vi "Set Initialization Data - TCP Send.vi"(8 "error in":errorcluster, 11 "Network End Point in":refnum<class "Network End Point.lvclass">) -> (0 "error out":errorcluster, 3 "Network End Point out":refnum<class "Network End Point.lvclass">)   [LabVIEW 2020, in "Network End Point.lvclass"]
doc: "Sets the initialization data of a statically linked subWorker."
uses:
  Network End Point.lvclass
  C:/Program Files (x86)/National Instruments/LabVIEW 2020/vi.lib/addons/_Workers/Library/Classes/Worker/Worker.lvclass
  TCP Send/Initialization Data.ctl
  <vilib>/addons/_Workers/Library/Classes/Message Queue/Message Queue.lvclass
  Network End Point.lvclass/Network End Point.ctl
  TCP Send/TCP Send.lvclass
  <vilib>/addons/_Workers/Library/Classes/Worker/Worker.lvclass
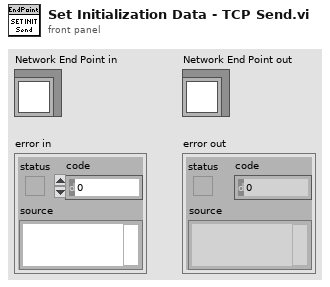
[diagram p1: front panel]
types:
  T1 = typedef "TCP Send.lvclass/Initialization Data.ctl" = cluster{"String":string, "connection ID":refnum<k5>, "End Point":refnum<class "Message Queue.lvclass">}
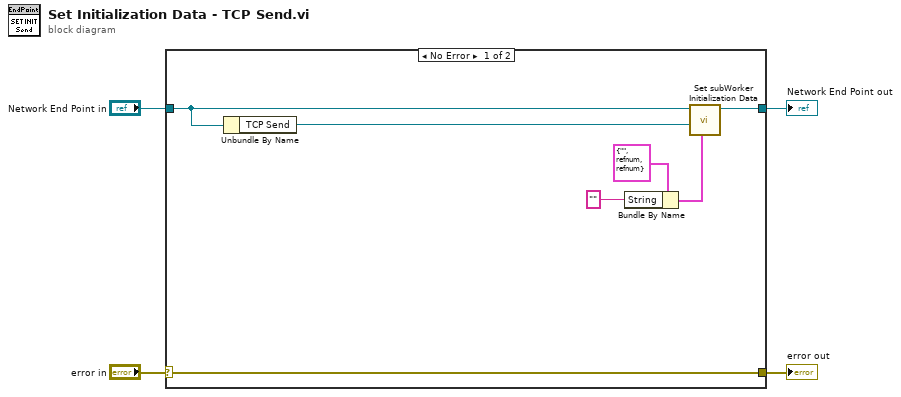
[diagram p0: block diagram]
diagram:
  n1 = case shown="No Error" "error in" {
    selector: "error in" -> [w11 w13]
    tunnel: [w11 w13] -> w3
    tunnel: [w9 w12] -> w2
    tunnel: "Network End Point in" -> [w8 w12]
    frame No Error {
      n2 = Unbundle By Name(w8) -> ("TCP Send"=w10:refnum<class "TCP Send.lvclass">)
      n3 = Bundle By Name(cluster=T1 {"String"="", "connection ID"=refnum, "End Point"=refnum} ("Initialization Data"), "String"="" ("Placeholder")) -> (w6:T1)
      n4 = call <vilib>:"Set subWorker Initialization Data.vi"("Initialization Data"=w6, "subWorker"=w10, "Worker"=w8) -> ("Worker out"=w9:refnum<class "Network End Point.lvclass">)  [unwired: 8 in]
    }
    frame Error {
    }
  }
  "error out" <- w3
  "Network End Point out" <- w2
